vi "Init Panels.vi"(8 "error in (no error)":errorcluster, 11 "App in":refnum<class "App.lvclass">) -> (0 "error out":errorcluster, 3 "App out":refnum<class "App.lvclass">)   [LabVIEW 2020, in "PicoG-App.lvlib" / "App.lvclass"]
uses:
  App.lvclass
  App.lvclass/App.ctl
  <vilib>/IlluminatedG/IG OOPanel/OOPanel/Manager/Manager.lvclass
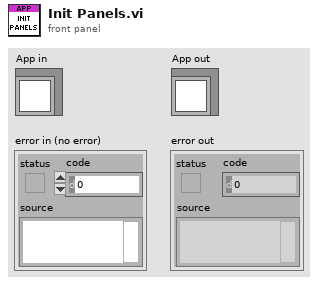
[diagram p1: front panel]
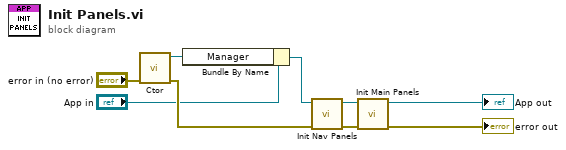
[diagram p0: block diagram]
diagram:
  n1 = call <vilib>:"Ctor.vi"("error in (no error)"="error in (no error)") -> ("error out"=w9:errorcluster, "Manager out"=w7:refnum<class "Manager.lvclass">)  [unwired: 9 in]
  n2 = Bundle By Name(cluster="App in", "Manager"=w7) -> (w2:refnum<class "App.lvclass">)
  n3 = call "Init Nav Panels.vi"("error in (no error)"=w9, "App in"=w2) -> ("error out"=w6:errorcluster, "App out"=w3:refnum<class "App.lvclass">)  [unwired: 8 in]
  n4 = call "Init Main Panels.vi"("error in (no error)"=w6, "App in"=w3) -> ("error out"=→"error out":errorcluster, "App out"=→"App out":refnum<class "App.lvclass">)  [unwired: 8 in]
